vi "Create Version VI Icon.vi"(7 "Library Ref":refnum<vi>, 8 "error in (no error)":errorcluster, 11 "VI Ref":refnum<vi>) -> (0 "error out":errorcluster, 3 "VI out":refnum<vi>)   [LabVIEW 2019]
doc: "Generates an icon with a border, the text layers \"GET VERSION\" (2 lines) and the NI_Library layer."
uses:
  <vilib>/LabVIEW Icon API/lv_icon/Classes/Icon/Icon.lvclass
  <vilib>/LabVIEW Icon API/API_User Layer Data.ctl
  <vilib>/Utility/miscctls.llb/LVPoint32TypeDef.ctl
  <vilib>/picture/picture.llb/imagedata.ctl
  <vilib>/LabVIEW Icon API/API_Text.ctl
  <vilib>/LabVIEW Icon API/LabVIEW Icon API.lvlib
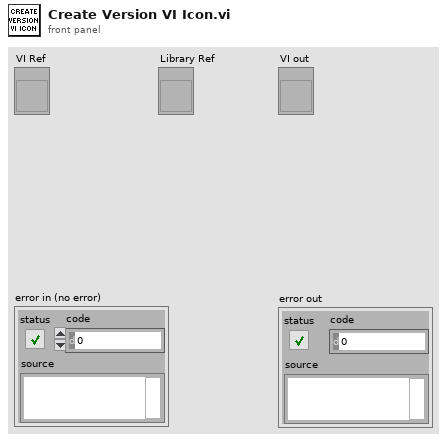
[diagram p1: front panel]
types:
  T1 = typedef "LabVIEW Icon API.lvlib/API_Text.ctl" = cluster{"Line 1 text":string, "Line 2 text":string, "Line 3 text":string, "Line 4 text":string}
  T2 = typedef "LabVIEW Icon API.lvlib/API_User Layer Data.ctl" = cluster{"Layer name":string, "Origin":T3, "Icon image data":T4}
  T3 = typedef "LVPoint32TypeDef.ctl" = cluster{"Horizontal":i32, "Vertical":i32}
  T4 = typedef "imagedata.ctl" = cluster{"image type":i32, "image depth":i32, "image":u8[], "mask":u8[], "colors":u32[], "Rectangle":cluster{"left":i16, "top":i16, "right":i16, "bottom":i16}}
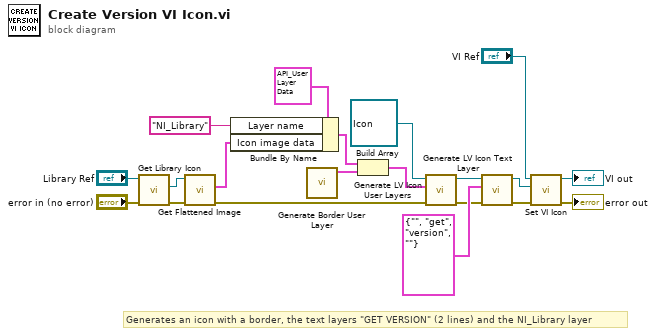
[diagram p0: block diagram]
diagram:
  # "Generates an icon with a border, the text layers \"GET VERSION\" (2 lines) and the NI_Library layer"
  n1 = call <vilib>:"Get Library Icon.vi"("error in (no error)"="error in (no error)", "Library Refnum in"="Library Ref") -> ("error out"=w5:errorcluster, "Icon"=w7:refnum<class "Icon.lvclass">)  [unwired: 7 in, 1 out]
  n2 = call <vilib>:"Get Flattened Image.vi"("error in (no error)"=w5, "lv_icon.lvlib:Icon.lvclass in"=w7) -> ("error out"=w4:errorcluster, "Color Image"=w12:T4)  [unwired: 6 in, 2 out]
  n3 = Bundle By Name(cluster=T2 {"Layer name"="", "Origin"={"Horizontal"=0, "Vertical"=0}, "Icon image data"={"image type"=0, "image depth"=0, "image"=[], "mask"=[], "colors"=[], "Rectangle"={"left"=0, "top"=0, "right"=0, "bottom"=0}}} ("User layer"), "Layer name"="NI_Library", "Icon image data"=w12) -> (w15:T2)
  n4 = call <vilib>:"Generate Border User Layer.vi"() -> ("User Layer data"=w14:T2)  [unwired: 11 in]
  n5 = Build Array(w15, w14) -> (w16:T2[])
  n6 = call <vilib>:"Generate LV Icon User Layers.vi"("error in (no error)"=w4, "User layers"=w16, "Icon in"=refnum<class "Icon.lvclass"> refnum ("Icon.lvclass")) -> ("error out"=w3:errorcluster, "Icon out"=w19:refnum<class "Icon.lvclass">)  [unwired: 7 in]
  n7 = call <vilib>:"Generate LV Icon Text Layer.vi"("error in (no error)"=w3, "Text"=T1 {"Line 1 text"="", "Line 2 text"="get", "Line 3 text"="version", "Line 4 text"=""}, "Icon in"=w19) -> ("error out"=w2:errorcluster, "Icon out"=w20:refnum<class "Icon.lvclass">)  [unwired: 7 in]
  n8 = call <vilib>:"Set VI Icon.vi"("error in (no error)"=w2, "Icon"=w20, "VI Refnum in"="VI Ref") -> ("error out"=→"error out":errorcluster, "VI Refnum out"=→"VI out":refnum<vi>)  [unwired: 7 in]
